vi "启动测量模式选择对话框.vi"(9 "量程选择":enum16{"L", "H", "AUTO"}(ring), 10 "启动选择":u16(ring) items=["水样测试", "标样核查", "零点核查", "跨度核查", "空白测试", "加标回收", "平行样", "校零", "校标"], 11 "确定":bool) -> (1 "标样浓度输出":dbl, 2 "量程选择输出":enum16{"L", "H", "AUTO"}(ring), 3 "启动选择输出":u16(ring) items=["水样测试", "标样核查", "零点核查", "跨度核查", "空白测试", "加标回收", "平行样", "校零", "校标"])   [LabVIEW 2016, in "斯坦道CODMn.lvlib"]
uses:
  <vilib>/Utility/miscctls.llb/LVPointTypeDef.ctl
panel:
  in  "标样浓度:":dbl
  in  "取消":bool
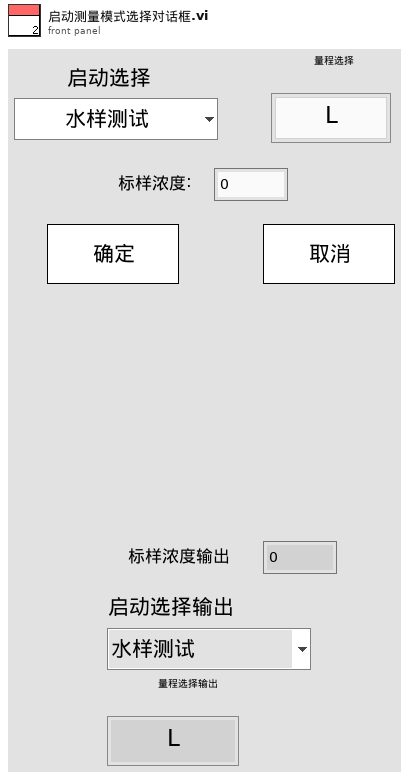
[diagram p1: front panel]
types:
  T1 = typedef "LVPointTypeDef.ctl" = cluster{"Horizontal":i16, "Vertical":i16}
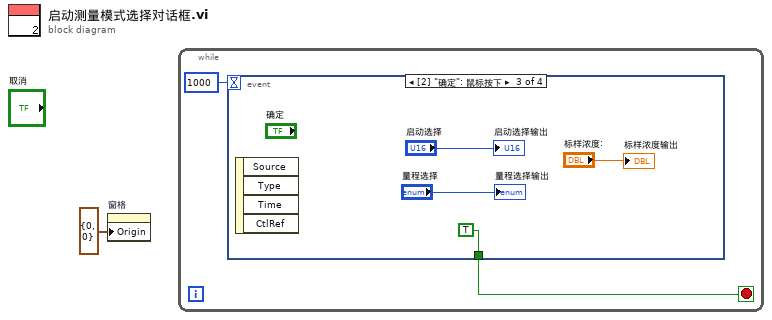
[diagram p0: block diagram]
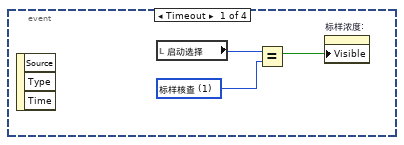
[diagram p2: hidden frame]
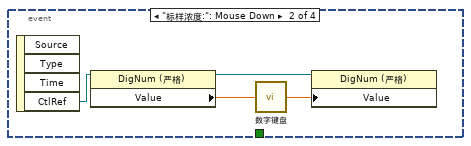
[diagram p3: hidden frame]
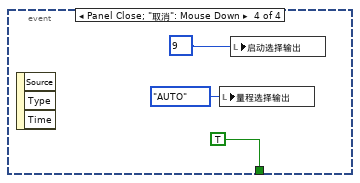
[diagram p4: hidden frame]
diagram:
  n1 = property on="窗格" class="Pane"("Origin"=T1 {"Horizontal"=0, "Vertical"=0} ("原点")) -> ()  [unwired: 2 in, 2 out]
  n2 = while {
    stop <- w3 stop-if-true
    n3 = event shown="[2] \"确定\": 鼠标按下" {
      selector: _ -> [_ _ _ _]
      dyn-events: _ -> [_ _ _ _]
      timeout: 1000 -> [_ _ _ _]
      tunnel: [_ _ TRUE TRUE] -> w3
      event Timeout {
        w5 = u16 1 items=["水样测试", "标样核查", "零点核查", "跨度核查", "空白测试", "加标回收", "平行样", "校零", "校标"] ("启动选择")
        n4 = event-data() -> ()  [unwired: 1 in, 3 out]
        n5 = local read "启动选择"() -> (w6:u16)
        n6 = Equal?(x=w6, y=w5) -> (x = y?=w4:bool)
        n7 = property on="标样浓度:" class="DigNum (严格)"("Visible"=w4) -> ()  [unwired: 2 in, 2 out]
      }
      event "标样浓度:": Mouse Down {
        n8 = event-data() -> ("CtlRef"=w10:refnum<vi>)  [unwired: 1 in, 3 out]
        n9 = property class="DigNum (严格)"(reference=w10) -> (reference out=w8:refnum<vi>, "Value"=w9:dbl)  [unwired: 1 in, 1 out]
        n10 = call "数字键盘.vi"("OldNumber"=w9) -> ("NewNumber"=w7:sgl)
        n11 = property class="DigNum (严格)"(reference=w8, "Value"=w7) -> ()  [unwired: 1 in, 2 out]
      }
      event "确定": Mouse Down {
        n12 = event-data() -> ()  [unwired: 1 in, 4 out]
        "启动选择输出" <- "启动选择"
        "量程选择输出" <- "量程选择"
        "标样浓度输出" <- "标样浓度:"
      }
      event Panel Close; "取消": Mouse Down {
        w16 = u16 9 items=["水样测试", "标样核查", "零点核查", "跨度核查", "空白测试", "加标回收", "平行样", "校零", "校标", ""] ("启动选择 2")
        n13 = event-data() -> ()  [unwired: 1 in, 3 out]
        n14 = local write "量程选择输出"(enum16{"L", "H", "AUTO"}."AUTO" ("量程选择输出")) -> ()
        n15 = local write "启动选择输出"(w16) -> ()
      }
    }
  }
